vi "Write name.vi"(8 "error in (no error)":errorcluster, 10 "name":string, 11 "Pizza":refnum<class "Pizza.lvclass">) -> (0 "error out":errorcluster, 3 "Pizza":refnum<class "Pizza.lvclass">)   [LabVIEW 2020, in "FactoryMethod.lvlib" / "PizzaFactoryMethod.lvlib" / "Pizza.lvclass"]
uses:
  Pizza.lvclass
  Pizza.lvclass/Pizza.ctl
  TypeDef/privateDataDVR.ctl
  TypeDef/privateData.ctl
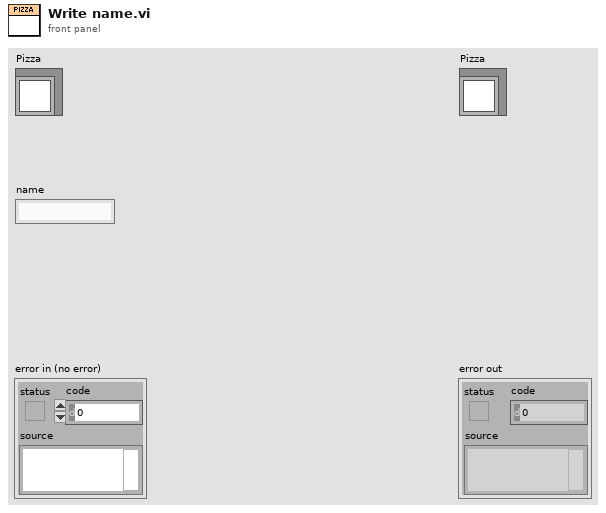
[diagram p1: front panel]
types:
  T1 = typedef "FactoryMethod.lvlib/PizzaFactoryMethod.lvlib/Pizza.lvclass/privateDataDVR.ctl" = refnum<data-value>
  T2 = typedef "FactoryMethod.lvlib/PizzaFactoryMethod.lvlib/Pizza.lvclass/privateData.ctl" = cluster{"name":string, "dough":string, "sauce":string, "toppings":string[]}
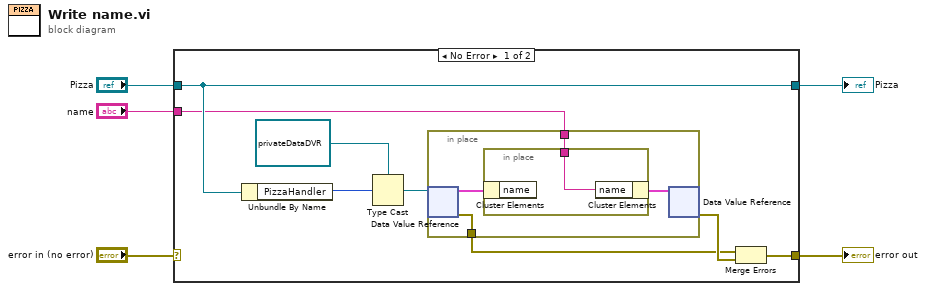
[diagram p0: block diagram]
diagram:
  n1 = case shown="No Error" "error in (no error)" {
    selector: "error in (no error)" -> [_ w20]
    tunnel: [w7 w20] -> w4
    tunnel: [w9 w19] -> w2
    tunnel: "Pizza" -> [w9 w19]
    tunnel: "name" -> [w6 _]
    frame No Error {
      n2 = Unbundle By Name(w9) -> ("PizzaHandler"=w11:u32)
      n3 = Type Cast(type=T1 refnum ("privateDataDVR"), x=w11) -> (*(type *) &x=w13:T1)
      n4 = in-place {
        in-place-border: [w16] -> w10
        in-place-border: w6 -> [w15]
        n5 = in-place-dvr #1(w13) -> (w17:T2, w16:errorcluster)
        n6 = in-place {
          in-place-border: w15 -> [w18]
          n7 = in-place-cluster #2(w17) -> ()  [unwired: 1 out]
          n8 = in-place-cluster #2("name"=w18) -> (w14:T2)
        }
        n9 = in-place-dvr #1(w14) -> (w12:errorcluster)  [unwired: 1 out]
      }
      n10 = Merge Errors(w10, w12) -> (w7:errorcluster)
    }
    frame Error {
    }
  }
  "error out" <- w4
  "Pizza" <- w2
